vi "testWriteArrayToFileAutoWrapInCluster.vi"(8 "error in (no error)":errorcluster, 11 "TestCase in":refnum<class "EasyXMLTest.lvclass">) -> (0 "error out":errorcluster, 3 "TestCase out":refnum<class "EasyXMLTest.lvclass">)   [LabVIEW 2011, in "EasyXMLTest.lvclass"]
doc: "Verify that error in is not overwritten"
uses:
  EasyXMLTest.lvclass
panel:
  in  "MyArray":string[](array[string])=["foo", "bar"]
  in  "Expected File Contents":string="<unnamed_cluster>\n  <MyArray>foo</MyArray>\n  <MyArray>bar</MyArray>\n</unnamed_cluster>"
  out "File Contents":string
  # "<== Write File input"
  # "<== Expected File"
  # "Actual File ==>"
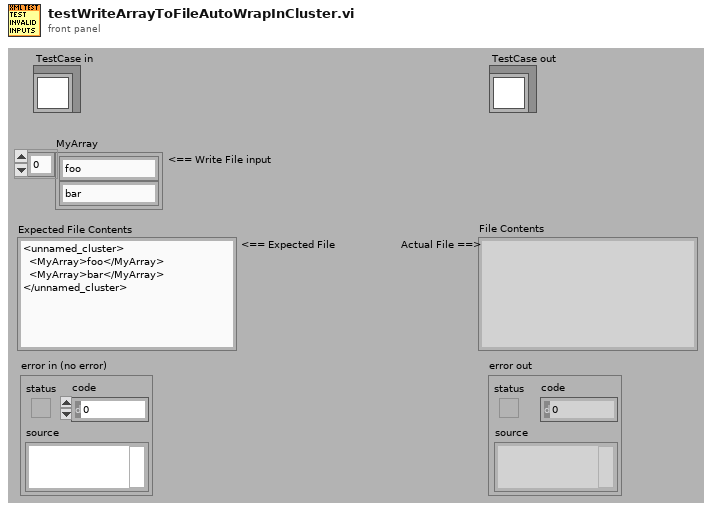
[diagram p1: front panel]
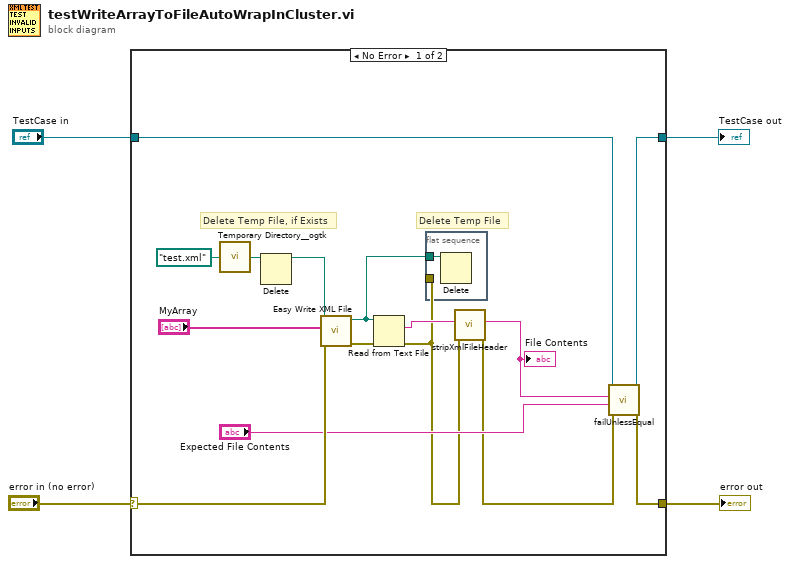
[diagram p0: block diagram]
diagram:
  n1 = case shown="No Error" "error in (no error)" {
    selector: "error in (no error)" -> [w18 w22]
    tunnel: [w9 w22] -> w3
    tunnel: [w10 w21] -> w1
    tunnel: "TestCase in" -> [w11 w21]
    frame No Error {
      # "Delete Temp File"
      # "Delete Temp File, if Exists"
      n2 = call <userlib>:"Temporary Directory__ogtk.vi"("Relative path (.)"=path "test.xml") -> ("Temporary Directory (+ Relative)"=w16:path)
      n3 = Delete(path (use dialog)=w16) -> (deleted path=w15:path)  [unwired: 4 in, 2 out]
      n4 = call "Easy Write XML File.vi"("error in (no error)"=w18, "LabVIEW Data"="MyArray", "XML File Path"=w15) -> ("error out"=w13:errorcluster, "XML File Path (duplicate)"=w14:path)  [unwired: 7 in]
      n5 = Read from Text File(file (use dialog)=w14, error in=w13) -> (text=w8:string, error out=w6:errorcluster)  [unwired: 2 in, 2 out]
      n6 = flat-sequence {
        tunnel: w14 -> [w20]
        tunnel: w6 -> [_]
        frame #0 {
          n7 = Delete(path (use dialog)=w20) -> ()  [unwired: 4 in, 3 out]
        }
      }
      n8 = call "stripXmlFileHeader.vi"("error in (no error)"=w6, "XML File String"=w8) -> ("error out"=w5:errorcluster, "XML File Document"=w7:string)  [unwired: 7 in, 1 out]
      "File Contents" <- w7
      n9 = call-dynamic "failUnlessEqual.vi"("error in (no error)"=w5, "y"="Expected File Contents", "x"=w7, "TestCase in"=w11) -> ("error out"=w9:errorcluster, "TestCase out"=w10:refnum<class "EasyXMLTest.lvclass">)  [unwired: 6 in]
    }
    frame Error {
    }
  }
  "error out" <- w3
  "TestCase out" <- w1
